vi "RMC解码.vi"(11 "所有匹配":string="014600.00,A,2237.496474,N,11356.089515,E,0.0,225.5,310518,2.3,W,A*23\r\n") -> (2 "经度":dbl, 3 "纬度":dbl, 5 "定位OK?":bool)   [LabVIEW 2016, in "GPS.lvlib" / "GPS.lvclass"]
uses:
  GPS.lvclass
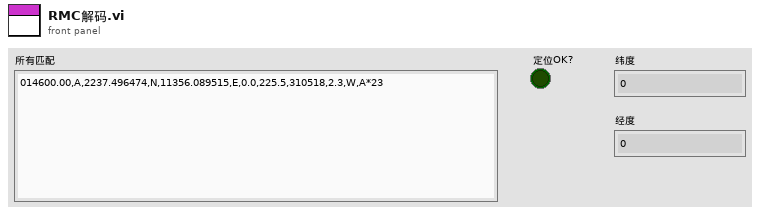
[diagram p1: front panel]
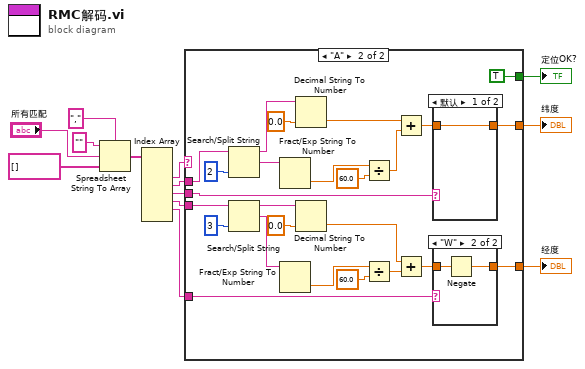
[diagram p0: block diagram]
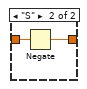
[diagram p4: hidden frame]
diagram:
  n1 = Spreadsheet String To Array(delimiter (Tab)="," ("分隔符(Tab)"), format string="" ("格式字符串"), spreadsheet string="所有匹配", array type (2D Dbl)=string[] [] ("数组类型(2D Dbl)")) -> (array=w9:string[])
  n2 = Index Array(array=w9) -> (element #2=w2:string, element #3=w7:string, element #4=w8:string, element #5=w4:string, element #6=w3:string)  [unwired: 7 in, 2 out]
  n3 = case shown="\"A\"" w2 {
    tunnel: w8 -> [_ w16]
    tunnel: w7 -> [_ w17]
    tunnel: [_ w29] -> w6
    tunnel: [_ w28] -> w5
    tunnel: w4 -> [_ w15]
    tunnel: w3 -> [_ w14]
    tunnel: [_ TRUE] -> w1
    frame Default {
    }
    frame "A" {
      n4 = Search/Split String(string=w17, offset (0)=2 ("偏移量(0)")) -> (substring before match=w34:string, match + rest of string=w37:string)  [unwired: 1 in, 1 out]
      n5 = Search/Split String(string=w15, offset (0)=3 ("偏移量(0)")) -> (substring before match=w23:string, match + rest of string=w20:string)  [unwired: 1 in, 1 out]
      n6 = Fract/Exp String To Number(string=w37) -> (number=w36:dbl)  [unwired: 3 in, 1 out]
      n7 = Fract/Exp String To Number(string=w20) -> (number=w21:dbl)  [unwired: 3 in, 1 out]
      n8 = Decimal String To Number(string=w34, default (0L)=0.0 ("默认(0 I32)")) -> (number=w32:dbl)  [unwired: 1 in, 1 out]
      n9 = Decimal String To Number(string=w23, default (0L)=0.0 ("默认(0 I32)")) -> (number=w25:dbl)  [unwired: 1 in, 1 out]
      n10 = Divide(x=w36, y=60.0) -> (x/y=w33:dbl)
      n11 = Divide(x=w21, y=60.0) -> (x/y=w24:dbl)
      n12 = Add(x=w32, y=w33) -> (x+y=w30:dbl)
      n13 = Add(x=w25, y=w24) -> (x+y=w27:dbl)
      n14 = case shown="默认" w16 {
        tunnel: w30 -> [w42 w44]
        tunnel: [w42 w43] -> w29
        frame Default {
        }
        frame "S" {
          n15 = Negate(x=w44) -> (-x=w43:dbl)
        }
      }
      n16 = case shown="\"W\"" w14 {
        tunnel: w27 -> [w39 w41]
        tunnel: [w39 w40] -> w28
        frame Default {
        }
        frame "W" {
          n17 = Negate(x=w41) -> (-x=w40:dbl)
        }
      }
    }
  }
  "纬度" <- w6
  "经度" <- w5
  "定位OK?" <- w1
